vi "CRD HF v2.vi"() -> (0 "error out":errorcluster)   [LabVIEW 2015]
uses:
  <vilib>/rvi/eio/common/nirviEmuClasses.ctl
  <vilib>/rvi/Emulation/niFpgaGetClockAttributes.vi
  <vilib>/rvi/Emulation/niFpgaSctlEmulationGetInTimedLoop.vi
  <vilib>/rvi/Emulation/niFpgaEmulationReportErrorSimple.vi
  <vilib>/rvi/Emulation/niFpgaEmulationIsFPGAContextNoSignature.vi
  <vilib>/rvi/DataTransferAndStorage/Container/Common/niFpgaContainerGetUniqueNameForEmu.vi
  <vilib>/rvi/Memory/Memory_Emulation/niFpgaMemoryEmulationCacheClearOnFirstRun.vi
  <vilib>/rvi/Memory/Memory_Emulation/nirvimemoryEmulationManagerCache_MakeExclusive.vi
  <vilib>/rvi/Memory/Memory_Emulation/niFpgaMemoryEmulationValidateCache.vi
  <vilib>/rvi/Memory/Memory_Emulation/nirvimemoryEmulationManagerCache_InsertValue.vi
  <vilib>/Utility/error.llb/Clear Errors.vi
  <vilib>/rvi/Memory/Memory_Emulation/nirvimemoryEmulationManagerCache_ReleaseExclusive.vi
  <vilib>/rvi/Memory/Memory_Emulation/nirvimemoryEmulationManagerCache_GetValue.vi
  <vilib>/rvi/Memory/Memory_Emulation/nirvimemoryEmulationManagerCache_SetValue.vi
  <vilib>/rvi/Emulation/niFpgaProcessEmulError.vi
  <vilib>/rvi/eio/common/nirviEmuTemplateMethod_errors.vi
  <vilib>/rvi/Emulation/niFpgaCriticalErrorInLSC.vi
  <vilib>/rvi/FIFO/Fifo_Resource/nirvififoEmulationSetSize.vi
  <vilib>/rvi/FIFO/Fifo_Resource/nirviFifoEmulationQueueMgr.vi
  <instcachedir>/0/nirviFifoEmulationQueueMgr_E5CAEC123FF24DC58D834DCA3CDAA9B5.lvgen/nirviFifoEmulationQueueMgr_E5CAEC123FF24DC58D834DCA3CDAA9B5_001.vi
  <vilib>/rvi/errors/niFpgaSetErrorForExecOnDevCompSimple.vi
  <vilib>/rvi/eio/common/nirviEmuReportErrorAndStop.vi
  <vilib>/rvi/FIFO/Fifo_Resource/nirvififoEmulationCreateLock.vi
  <vilib>/rvi/FIFO/Fifo_Resource/nirvififoEmulationObtainLock.vi
  <vilib>/rvi/FIFO/Fifo_Resource/nirvififoEmulationReleaseLock.vi
  <vilib>/rvi/occurrence/nirviWaitOnOccurrenceBase.vi
  <vilib>/rvi/errors/nirviReportUnexpectedCaseInternalError.vi
  <vilib>/rvi/errors/nirviReportUnexpectedCaseInternalError (U32).vi
  <vilib>/rvi/DataTransferAndStorage/Container/Common/niFpgaContainerExecOnDevCompGetState.vi
  <vilib>/rvi/FIFO/Fifo_Resource/nirvififoEmulationDetermineInputValidOut.vi
  <vilib>/rvi/interface/RandomDataEmulation/niFpgaRandomDataHandleErrors.vi
  <vilib>/rvi/Memory/Memory_Emulation/nirvimemoryFastEmulation.vi
  <vilib>/rvi/Memory/Memory_Emulation/nirvimemoryEmulation.vi
  <vilib>/rvi/DataTransferAndStorage/Container/XNode/niFpgaContainer.xnode
  <vilib>/rvi/DataTransferAndStorage/Register/Emulation/niFpgaRegisterEmulation.vi
  <vilib>/eio/EIOGrowableMethodNode/genericMethod/EIOGrowableMethodNode.xnode
  <vilib>/rvi/eio/nirviEIOMethodImplementation/nirviEIOMethodImplementation.xnode
  <vilib>/rvi/eio/nirviErrorMerge/nirviErrorMerge.xnode
  <vilib>/rvi/FIFO/Fifo_Resource/nirvififoEmulationGetNumberOfElementsToRead.vi
  <vilib>/rvi/FIFO/Fifo_Resource/nirvififoEmulationRead.vi
  <vilib>/rvi/FIFO/Fifo_Resource/niFpgaFifoEmulationRefIn.vi
  <vilib>/rvi/FXPMathLib/FxpAdd/XNode/nifxpmath_Add.xnode
  <vilib>/rvi/interface/RandomDataEmulation/nirviRandomDataFpgaReadWriteTemplate.vi
  <vilib>/rvi/FXPMathLib/FxpSub/XNode/nifxpmath_Sub.xnode
  <vilib>/eio/EIONode/EIONode.xnode
  <vilib>/rvi/FIFO/Fifo_Resource/nirvififoEmulationWrite.vi
  <vilib>/rvi/FXPMathLib/sim/FxpSim.dll
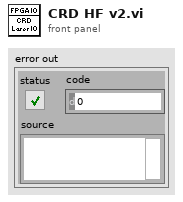
[diagram p1: front panel]
types:
  T1 = typedef "nirviEmuClasses.ctl" = enum16{"IO Read", "IO Write", "Method", "Property Read", "Property Write"}
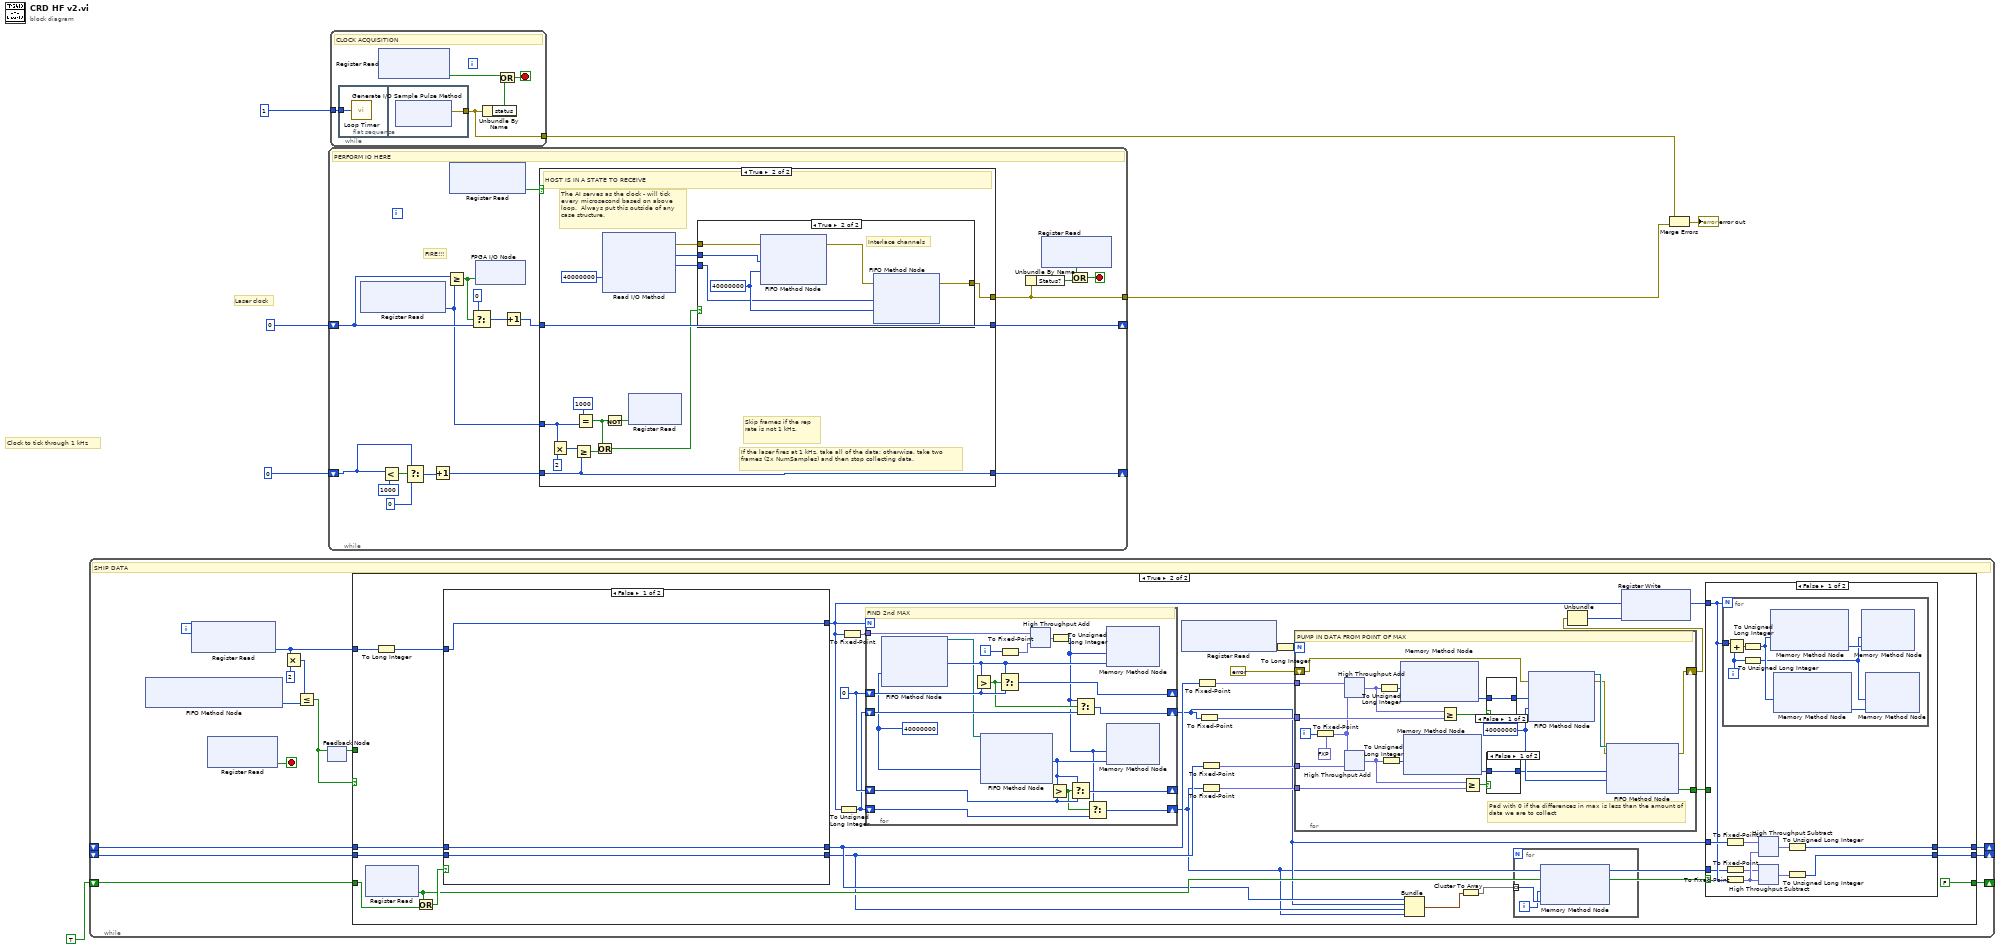
[diagram p0: block diagram]
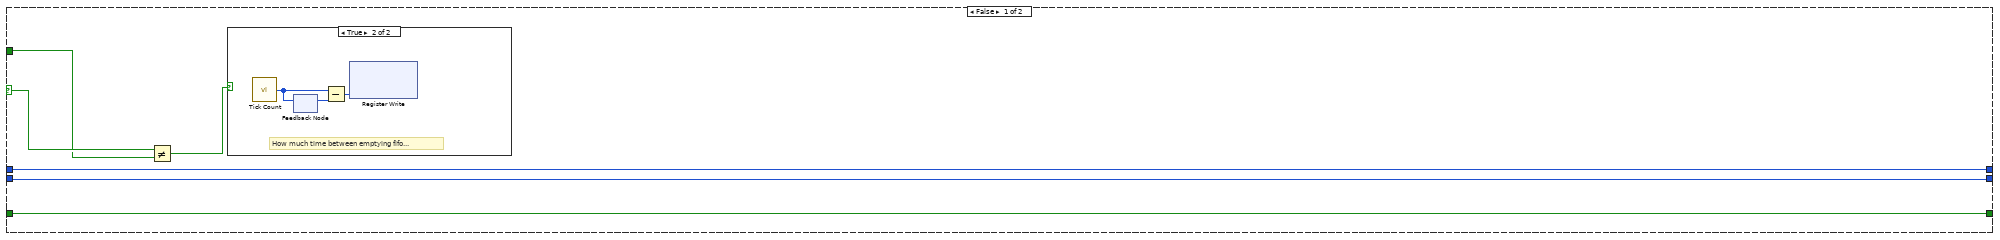
[diagram p2: hidden frame]
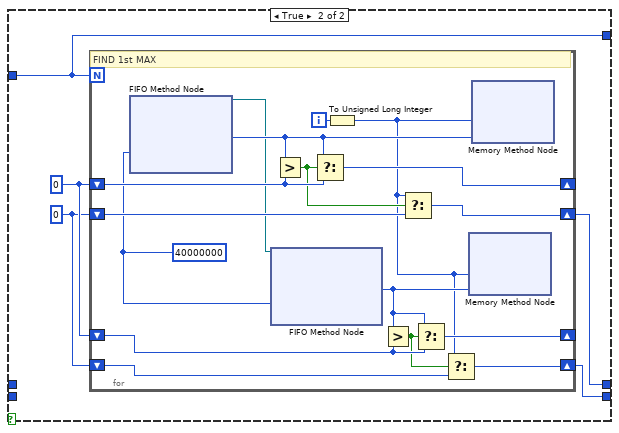
[diagram p5: hidden frame]
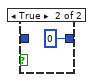
[diagram p6: hidden frame]
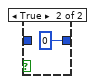
[diagram p7: hidden frame]
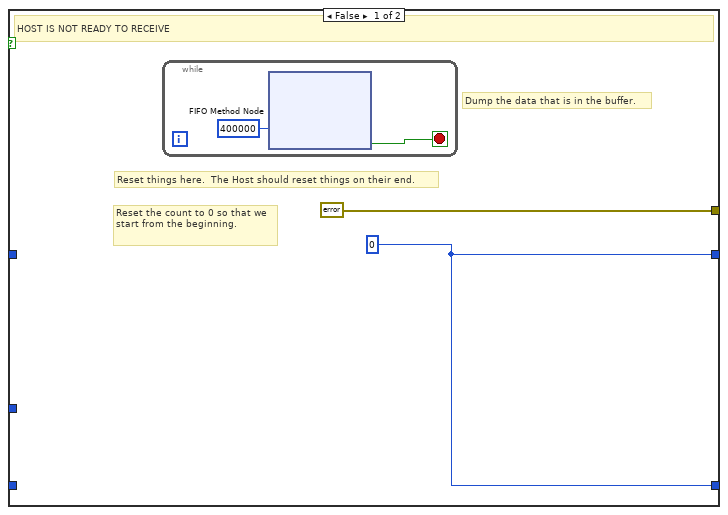
[diagram p8: hidden frame]
diagram:
  # "Laser clock"
  # "Clock to tick through 1 kHz"
  n1 = while {
    shift-right: [w18] -> _
    shift-left: _ -> [w20]
    shift-right: [w17] -> _
    shift-left: _ -> [w19]
    shift-right: [w15] -> _
    shift-left: TRUE -> [w16]
    stop <- w10 stop-if-true
    # "SHIP DATA"
    n2 = xnode ("FIFO Method Node")() -> ("Number of Elements to Read"=w11:u32)  [unwired: 2 in, 2 out]
    n3 = xnode ("Register Read")() -> ("Data"=w14:u16)  [unwired: 1 in, 1 out]
    n4 = xnode ("Register Read")() -> ("Data"=w10:bool)  [unwired: 1 in, 1 out]
    n5 = Multiply(x=w14, y=u16 2) -> (x*y=w12:u16)
    n6 = Less Or Equal?(x=w12, y=w11) -> (x <= y?=w9:bool)
    n7 = feedback-in #1(w9) -> ()
    n8 = feedback #1() -> (w8:bool)  [unwired: 1 in]
    n9 = case shown="True" w9 {
      selector: w9 -> [w23 _]
      tunnel: w14 -> [_ w59]
      tunnel: w20 -> [w26 w57]
      tunnel: w19 -> [w25 w56]
      tunnel: [w26 w55] -> w18
      tunnel: [w25 w54] -> w17
      tunnel: w16 -> [w24 w47]
      tunnel: [w24 FALSE] -> w15
      tunnel: w8 -> [w22 _]
      frame False {
        n10 = Not Equal?(x=w23, y=w22) -> (x != y?=w21:bool)
        n11 = case shown="True" w21 {
          frame False {
          }
          frame True {
            # "How much time between emptying fifo..."
            n12 = call "Tick Count"() -> ("Tick Count(Ticks)"=w28:u32)
            n13 = feedback #2() -> (w27:u32)  [unwired: 1 in]
            n14 = feedback-in #2(w28) -> ()
            n15 = Subtract(x=w28, y=w27) -> (x-y=w29:u32)
            n16 = xnode ("Register Write")("Data"=w29) -> ()  [unwired: 1 in, 1 out]
          }
        }
      }
      frame True {
        w53 = i16 0 ("Element")
        n17 = xnode ("Register Read")() -> ("Data"=w45:bool)  [unwired: 1 in, 1 out]
        n18 = To Long Integer(number=w59) -> (32bit integer=w50:i32)
        n19 = Or(x=w45, y=w47) -> (x .or. y?=w46:bool)
        n20 = case shown="False" w46 {
          tunnel: [w80 w86] -> w37
          tunnel: [w81 w85] -> w39
          tunnel: w50 -> [w79 w82]
          tunnel: w57 -> [w81 _]
          tunnel: w56 -> [w80 _]
          tunnel: [w79 w82] -> w30
          frame False {
          }
          frame True {
            w83 = u32 0 ("Element")
            w84 = i16 0 ("Element")
            n21 = for {
              N: w82 -> [_]
              shift-right: [w100] -> _
              shift-left: w84 -> [w101]
              shift-right: [w97] -> w85
              shift-left: w83 -> [w98]
              shift-right: [w89] -> w86
              shift-left: w83 -> [w90]
              shift-right: [w94] -> _
              shift-left: w84 -> [w93]
              i -> [w91]
              w88 = 40000000 ("Timeout")
              # "FIND 1st MAX"
              n22 = xnode ("FIFO Method Node")("Timeout"=w88) -> ("Element"=w102:i16, "FIFO Out"=w96:refnum<k21>)  [unwired: 1 in, 1 out]
              n23 = xnode ("FIFO Method Node")("Timeout"=w88, "FIFO In"=w96) -> ("Element"=w95:i16)  [unwired: 2 out]
              n24 = Greater?(x=w102, y=w101) -> (0:w99:bool)
              n25 = Select(t=w102, s=w99, f=w101) -> (s? t:f=w100:i16)
              n26 = To Unsigned Long Integer(number=w91) -> (unsigned 32bit integer=w87:u32)
              n27 = Greater?(x=w95, y=w93) -> (0:w92:bool)
              n28 = Select(t=w87, s=w99, f=w98) -> (s? t:f=w97:u32)
              n29 = Select(t=w95, s=w92, f=w93) -> (s? t:f=w94:i16)
              n30 = Select(t=w87, s=w92, f=w90) -> (s? t:f=w89:u32)
              n31 = xnode ("Memory Method Node")("Address"=w87, "Data"=w95) -> ()  [unwired: 1 in, 1 out]
              n32 = xnode ("Memory Method Node")("Address"=w87, "Data"=w102) -> ()  [unwired: 1 in, 1 out]
            }
          }
        }
        n33 = To Unsigned Long Integer(number=w30) -> (unsigned 32bit integer=w52:u32)
        n34 = To Fixed-Point(number=w30) -> (fixed-point=w51:fxp<+/-,32,32>)  [unwired: 1 in]
        n35 = for {
          N: w30 -> [_]
          shift-right: [w146] -> _
          shift-left: w53 -> [w147]
          shift-right: [w143] -> w38
          shift-left: w52 -> [w144]
          shift-right: [w136] -> w36
          shift-left: w52 -> [w137]
          shift-right: [w140] -> _
          shift-left: w53 -> [w139]
          tunnel: w51 -> [w132]
          i -> [w133]
          w135 = 40000000 ("Timeout")
          # "FIND 2nd MAX"
          n36 = xnode ("FIFO Method Node")("Timeout"=w135) -> ("Element"=w148:i16, "FIFO Out"=w142:refnum<k21>)  [unwired: 1 in, 1 out]
          n37 = Greater?(x=w148, y=w147) -> (0:w145:bool)
          n38 = xnode ("FIFO Method Node")("Timeout"=w135, "FIFO In"=w142) -> ("Element"=w141:i16)  [unwired: 2 out]
          n39 = Select(t=w148, s=w145, f=w147) -> (s? t:f=w146:i16)
          n40 = To Fixed-Point(number=w133) -> (fixed-point=w131:fxp<+/-,32,32>)  [unwired: 1 in]
          n41 = xnode ("High Throughput Add")("x"=w132, "y"=w131) -> ("x+y"=w130:fxp<+,32,32>)
          n42 = Greater?(x=w141, y=w139) -> (0:w138:bool)
          n43 = To Unsigned Long Integer(number=w130) -> (unsigned 32bit integer=w134:u32)
          n44 = Select(t=w141, s=w138, f=w139) -> (s? t:f=w140:i16)
          n45 = Select(t=w134, s=w145, f=w144) -> (s? t:f=w143:u32)
          n46 = Select(t=w134, s=w138, f=w137) -> (s? t:f=w136:u32)
          n47 = xnode ("Memory Method Node")("Address"=w134, "Data"=w148) -> ()  [unwired: 1 in, 1 out]
          n48 = xnode ("Memory Method Node")("Address"=w134, "Data"=w141) -> ()  [unwired: 1 in, 1 out]
        }
        n49 = xnode ("Register Read")() -> ("Data"=w42:u16)  [unwired: 1 in, 1 out]
        n50 = To Fixed-Point(number=w39) -> (fixed-point=w49:fxp<+,32,32>)  [unwired: 1 in]
        n51 = To Fixed-Point(number=w38) -> (fixed-point=w41:fxp<+,32,32>)  [unwired: 1 in]
        n52 = To Fixed-Point(number=w37) -> (fixed-point=w48:fxp<+,32,32>)  [unwired: 1 in]
        n53 = To Fixed-Point(number=w36) -> (fixed-point=w40:fxp<+,32,32>)  [unwired: 1 in]
        n54 = To Long Integer(number=w42) -> (32bit integer=w43:i32)
        n55 = for {
          N: w43 -> [_]
          tunnel: [w122] -> w58
          tunnel: w41 -> [w120]
          tunnel: w49 -> [w113]
          tunnel: w48 -> [w108]
          tunnel: w40 -> [w109]
          shift-right: [w104] -> w34
          shift-left: errorcluster {"Status?"=FALSE, "Code"=0, "Source"=""} ("error out") -> [w103]
          i -> [w111]
          w123 = 40000000 ("Timeout")
          # "Pad with 0 if the differences in max is less than the amount of data we are to collect"
          # "PUMP IN DATA FROM POINT OF MAX"
          n56 = To Fixed-Point(fixed-point type=fxp<+,32,32> 0.0, number=w111) -> (fixed-point=w112:fxp<+,32,32>)
          n57 = xnode ("High Throughput Add")("x"=w113, "y"=w112) -> ("x+y"=w110:fxp<+,32,32>)
          n58 = xnode ("High Throughput Add")("x"=w112, "y"=w108) -> ("x+y"=w107:fxp<+,32,32>)
          n59 = To Unsigned Long Integer(number=w110) -> (unsigned 32bit integer=w125:u32)
          n60 = To Unsigned Long Integer(number=w107) -> (unsigned 32bit integer=w121:u32)
          n61 = xnode ("Memory Method Node")("Address"=w125) -> ("Data"=w118:i16)  [unwired: 1 in, 1 out]
          n62 = xnode ("Memory Method Node")("Address"=w121) -> ("Data"=w115:i16)  [unwired: 1 in, 1 out]
          n63 = Greater Or Equal?(x=w110, y=w120) -> (x >= y?=w119:bool)
          n64 = Greater Or Equal?(x=w107, y=w109) -> (x >= y?=w116:bool)
          n65 = case shown="False" w119 {
            tunnel: w118 -> [w128 _]
            tunnel: [w128 i16 0 ("Data")] -> w117
            frame False {
            }
            frame True {
            }
          }
          n66 = case shown="False" w116 {
            tunnel: w115 -> [w126 _]
            tunnel: [w126 i16 0 ("Data")] -> w114
            frame False {
            }
            frame True {
            }
          }
          n67 = xnode ("FIFO Method Node")("Element"=w117, "Timeout"=w123, "error in (no error)"=w103) -> ("error out"=w105:errorcluster, "FIFO Out"=w124:refnum<k21>)  [unwired: 1 in, 1 out]
          n68 = xnode ("FIFO Method Node")("Element"=w114, "Timeout"=w123, "error in (no error)"=w105, "FIFO In"=w124) -> ("Timed Out?"=w122:bool, "error out"=w104:errorcluster)  [unwired: 1 out]
        }
        n69 = Bundle("Element"=w39, w38, "Element"=w37, w36) -> (w32:cluster{"Element":u32, u32, "Element":u32, u32})  [unwired: 1 in]
        n70 = Cluster To Array(cluster=w32) -> (array=w31:u32[])
        n71 = for {
          tunnel: w31 -> [w61] mode=indexing
          i -> [w60]
          n72 = xnode ("Memory Method Node")("Address"=w60, "Data"=w61) -> ()  [unwired: 1 in, 1 out]
        }
        n73 = Unbundle(w34) -> ("Code"=w33:i32)  [unwired: 2 out]
        n74 = xnode "Register Write"("Data"=w33) -> ()  [unwired: 1 in, 1 out]
        n75 = case shown="False" w45 {
          tunnel: w58 -> [_ _]
          tunnel: [w69 _] -> w55
          tunnel: [w65 _] -> w54
          tunnel: w38 -> [w64 _]
          tunnel: w30 -> [w63 _]
          tunnel: w36 -> [w62 _]
          frame False {
            n76 = for {
              N: w63 -> [_]
              tunnel: w63 -> [w78]
              i -> [w73]
              n77 = Add(x=w78, y=w73) -> (x+y=w75:i32)
              n78 = To Unsigned Long Integer(number=w75) -> (unsigned 32bit integer=w74:u32)
              n79 = To Unsigned Long Integer(number=w73) -> (unsigned 32bit integer=w72:u32)
              n80 = xnode ("Memory Method Node")("Address"=w74) -> ("Data"=w77:i16)  [unwired: 1 in, 1 out]
              n81 = xnode ("Memory Method Node")("Address"=w74) -> ("Data"=w76:i16)  [unwired: 1 in, 1 out]
              n82 = xnode ("Memory Method Node")("Address"=w72, "Data"=w77) -> ()  [unwired: 1 in, 1 out]
              n83 = xnode ("Memory Method Node")("Address"=w72, "Data"=w76) -> ()  [unwired: 1 in, 1 out]
            }
            n84 = To Fixed-Point(number=w64) -> (fixed-point=w71:fxp<+,32,32>)  [unwired: 1 in]
            n85 = To Fixed-Point(number=w62) -> (fixed-point=w67:fxp<+,32,32>)  [unwired: 1 in]
            n86 = To Fixed-Point(number=w63) -> (fixed-point=w68:fxp<+/-,32,32>)  [unwired: 1 in]
            n87 = xnode "High Throughput Subtract"("x"=w71, "y"=w68) -> ("x-y"=w70:fxp<+,32,32>)
            n88 = xnode "High Throughput Subtract"("x"=w67, "y"=w68) -> ("x-y"=w66:fxp<+,32,32>)
            n89 = To Unsigned Long Integer(number=w70) -> (unsigned 32bit integer=w69:u32)
            n90 = To Unsigned Long Integer(number=w66) -> (unsigned 32bit integer=w65:u32)
          }
          frame True {
          }
        }
      }
    }
  }
  n91 = while {
    shift-right: [w161] -> _
    shift-left: u16 0 ("Number of Samples") -> [w162]
    tunnel: [w165] -> w3
    shift-right: [w152] -> _
    shift-left: u16 0 ("Number of Samples") -> [w149]
    stop <- w151 stop-if-true
    # "FIRE!!!"
    # "PERFORM IO HERE"
    n92 = xnode ("Register Read")() -> ("Data"=w155:u16)  [unwired: 1 in, 1 out]
    n93 = Less?(x=w149, y=u16 1000) -> (x < y?=w154:bool)
    n94 = Select(t=w149, s=w154, f=u16 0 ("Number of Samples")) -> (s? t:f=w157:u16)
    n95 = Increment(x=w157) -> (x+1=w153:u16)
    n96 = Greater Or Equal?(x=w162, y=w155) -> (x >= y?=w164:bool)
    n97 = xnode ("Register Read")() -> ("Data"=w158:bool)  [unwired: 1 in, 1 out]
    n98 = Select(t=u16 0 ("Number of Samples"), s=w164, f=w162) -> (s? t:f=w160:u16)
    n99 = xnode "FPGA I/O Node"("CRDS"=w164) -> ()  [unwired: 1 in, 1 out]
    n100 = Increment(x=w160) -> (x+1=w159:u16)
    n101 = case shown="True" w158 {
      tunnel: [errorcluster {"Status?"=FALSE, "Code"=0, "Source"=""} ("error out") w172] -> w165
      tunnel: w159 -> [_ w186]
      tunnel: [w168 w186] -> w161
      tunnel: w155 -> [_ w182]
      tunnel: w153 -> [_ w177]
      tunnel: [w168 w177] -> w152
      frame False {
        w168 = u16 0 ("Number of Samples")
        # "Dump the data that is in the buffer."
        # "Reset things here.  The Host should reset things on their end."
        # "Reset the count to 0 so that we start from the beginning."
        # "HOST IS NOT READY TO RECEIVE"
        n102 = while {
          stop <- w171 stop-if-true
          n103 = xnode ("FIFO Method Node")("Timeout"=400000) -> ("Timed Out?"=w171:bool)  [unwired: 1 in, 2 out]
        }
      }
      frame True {
        # "The AI serves as the clock - will tick every microsecond based on above loop.  Always put this outside of any case structure."
        # "Skip frames if the rep rate is not 1 kHz."
        # "If the laser fires at 1 kHz, take all of the data; otherwise, take two frames (2x NumSamples) and then stop collecting data."
        # "HOST IS IN A STATE TO RECEIVE"
        n104 = Multiply(x=w182, y=u16 2) -> (x*y=w180:u16)
        n105 = Greater Or Equal?(x=w180, y=w177) -> (x >= y?=w179:bool)
        n106 = Equal?(x=u16 1000, y=w182) -> (x = y?=w184:bool)
        n107 = Or(x=w184, y=w179) -> (x .or. y?=w178:bool)
        n108 = xnode "Read I/O Method"("Timeout"=40000000) -> ("error out"=w174:errorcluster, "CRD Las Ch 1"=w175:i16, "CRD Las Ch 2"=w173:i16)  [unwired: 3 in, 3 out]
        n109 = Not(x=w184) -> (.not. x?=w183:bool)
        n110 = xnode ("Register Read")("Data"=w183) -> ()  [unwired: 1 in, 1 out]
        n111 = case shown="True" w178 {
          tunnel: w175 -> [_ w301]
          tunnel: w174 -> [w295 w300]
          tunnel: w173 -> [_ w298]
          tunnel: [w295 w296] -> w172
          frame False {
          }
          frame True {
            w299 = 40000000 ("Timeout")
            # "Interlace channels"
            n112 = xnode ("FIFO Method Node")("Element"=w301, "Timeout"=w299, "error in (no error)"=w300) -> ("error out"=w297:errorcluster)  [unwired: 1 in, 2 out]
            n113 = xnode ("FIFO Method Node")("Element"=w298, "Timeout"=w299, "error in (no error)"=w297) -> ("error out"=w296:errorcluster)  [unwired: 1 in, 2 out]
          }
        }
      }
    }
    n114 = Unbundle By Name(w165) -> ("Status?"=w167:bool)
    n115 = xnode ("Register Read")() -> ("Data"=w163:bool)  [unwired: 1 in, 1 out]
    n116 = Compound Arithmetic op=OR(w163, w167) -> (w151:bool)
  }
  n117 = while {
    tunnel: u32 1 ("Sample Period (uSec)") -> [w306]
    tunnel: [w305] -> w7
    stop <- w302 stop-if-true
    # "CLOCK ACQUISITION"
    n118 = flat-sequence {
      tunnel: w306 -> [w307]
      tunnel: [w308] -> w305
      frame #0 {
        n119 = call "Loop Timer"("Count(uSec)"=w307) -> ()  [unwired: 1 out]
      }
      frame #1 {
        n120 = xnode "Generate I/O Sample Pulse Method"() -> ("error out"=w308:errorcluster)  [unwired: 2 in, 1 out]
      }
    }
    n121 = xnode ("Register Read")() -> ("Data"=w304:bool)  [unwired: 1 in, 1 out]
    n122 = Unbundle By Name(w305) -> ("status"=w303:bool)
    n123 = Or(x=w304, y=w303) -> (x .or. y?=w302:bool)
  }
  n124 = Merge Errors(w7, w3) -> (→"error out":errorcluster)
